vi "Init Queues.vi"(8 "error in (no error)":errorcluster) -> (0 "error out":errorcluster, 3 "Queue Refs":T1)   [LabVIEW 2020, in "Queues.lvlib"]
doc: "Copyright 2015, 2016, 2017 National Instruments Corporation\n\nLicensed under the Apache License, Version 2.0 (the \"License\"); you may not use this file except in compliance with the License.\n\n You may obtain a copy of the License at\n\n http://www.apache.org/licenses/LICENSE-2.0\n\nUnless required by applicable law or agreed to in writing, software distributed under the License is distributed on an \"AS IS\" BASIS, WITHOUT WARRANTIES OR CONDITIONS OF ANY KIND, either express or implied.\n\nSee the License for the specific language governing permissions and limitations under the License."
uses:
  Queues.lvlib
  Queue Refs.ctl
  InterProcessQueueCtl.ctl
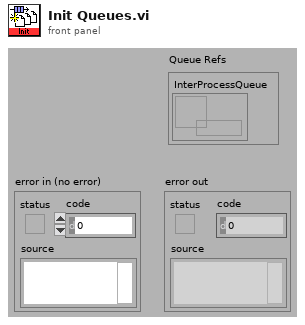
[diagram p1: front panel]
types:
  T1 = typedef "Queues.lvlib/Queue Refs.ctl" = cluster{"InterProcessQueue":refnum<queue>}
  T2 = typedef "Queues.lvlib/InterProcessQueueCtl.ctl" = cluster{"Command":string, "Data":variant}
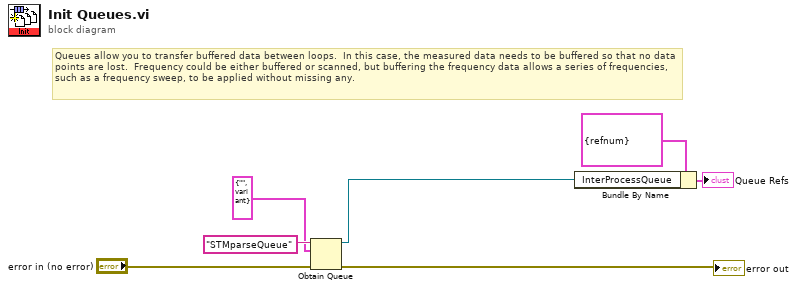
[diagram p0: block diagram]
diagram:
  # "Queues allow you to transfer buffered data between loops.  In this case, the measured data needs to be buffered so that no data points are lost.  Frequency could be either buffered or scanned, but buffering the frequency data allows a series of frequencies, such as a frequency sweep, to be applied without missing any."
  n1 = Obtain Queue(name (unnamed)="STMparseQueue", element data type=T2 {"Command"="", "Data"=variant} ("STMparseQueue"), error in (no error)="error in (no error)") -> (queue out=w4:refnum<queue>, error out=→"error out":errorcluster)  [unwired: 2 in, 1 out]
  n2 = Bundle By Name(cluster=T1 {"InterProcessQueue"=refnum} ("Queue Refs"), "InterProcessQueue"=w4) -> (→"Queue Refs":T1)
